vi "Read Config File (SubVI).vi"(0 "configuration file path":path=path "C:/Projet_CETAL_DESY_CSCI/POSTES LOCAUX/PROJECT_GAIA_HP/Development/Config/User.ini" caption="chemin du fichier de configuration", 5 "entrée d'erreur (pas d'erreur)":errorcluster) -> (14 "file path":path, 15 "User file contents Watlow":dbl[](array[numeric]), 18 "error?":bool caption="erreur ?", 19 "sortie d'erreur":errorcluster)   [LabVIEW 2017]
doc: "by Tanguy BOULARD"
uses:
  <vilib>/Utility/config.llb/Read Key (String).vi
  <vilib>/Utility/config.llb/NI_LVConfig.lvlib
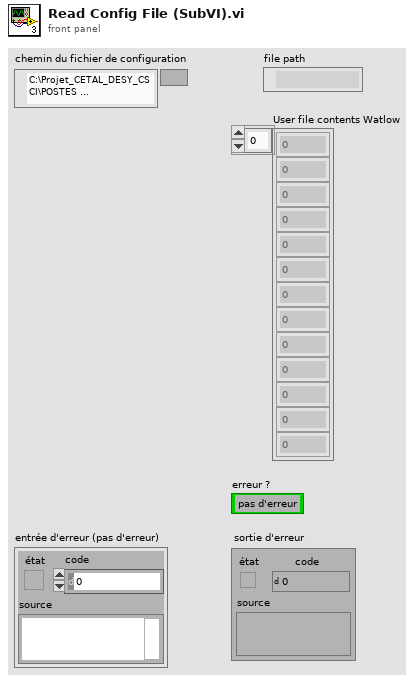
[diagram p1: front panel]
types:
  T1 = typedef "NI_LVConfig.lvlib/Config Data RefNum.ctl" = refnum<k1>
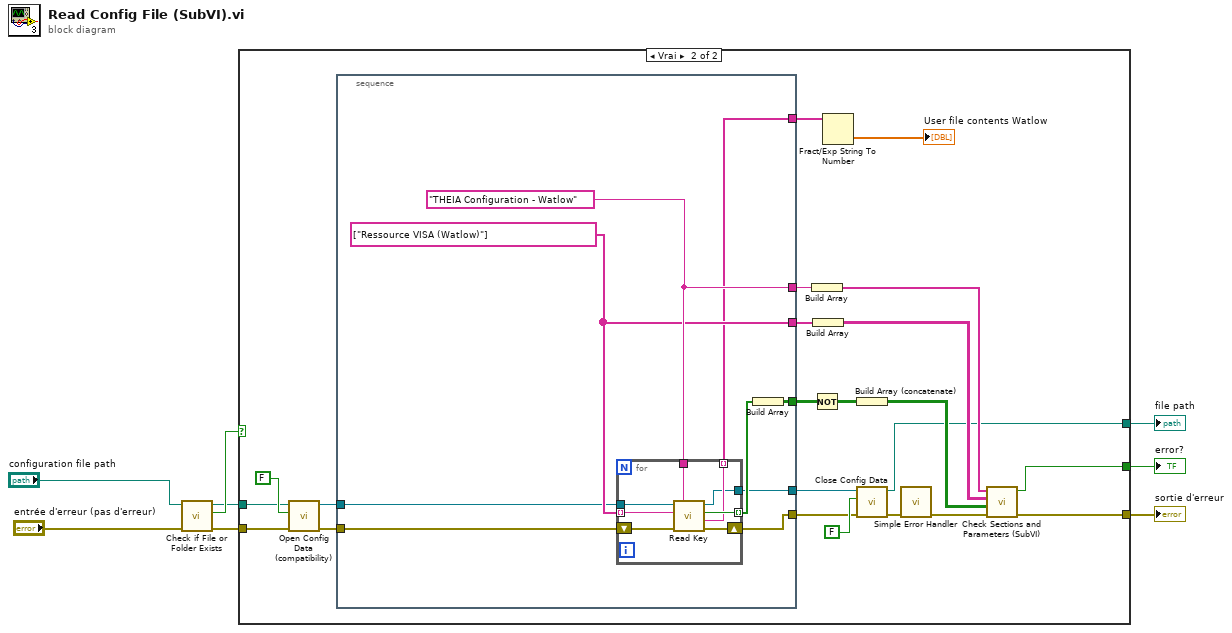
[diagram p0: block diagram]
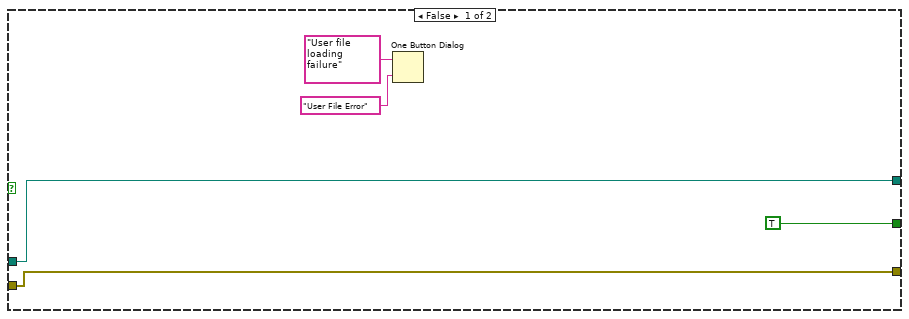
[diagram p2: hidden frame]
diagram:
  n1 = call <vilib>:"Check if File or Folder Exists.vi"("error in (no error)"="entrée d'erreur (pas d'erreur)", "path"="configuration file path") -> ("error out"=w5:errorcluster, "file or folder exists?"=w8:bool, "dup path"=w6:path)  [unwired: 7 in]
  n2 = case shown="Vrai" w8 {
    tunnel: w6 -> [w9 w31]
    tunnel: w5 -> [w11 w28]
    tunnel: [w11 w23] -> w3
    tunnel: [TRUE ("Erreur ?") w22] -> w4
    tunnel: [w9 w15] -> w1
    frame False {
      n3 = One Button Dialog(message="User file loading failure" ("Line1_message"), button name ("OK")="User File Error" ("Title")) -> ()  [unwired: 1 out]
    }
    frame True {
      n4 = call <vilib>:"Open Config Data (compatibility).vi"("error in (no error)"=w28, "create file if necessary (T)"=FALSE ("create file if necessary? (T)"), "configuration file path"=w31) -> ("error out"=w34:errorcluster, "refnum"=w29:T1)  [unwired: 6 in, 1 out]
      n5 = stacked-sequence {
        tunnel: w34 -> [w44]
        tunnel: w29 -> [w40]
        tunnel: [w37] -> w30
        tunnel: [w43] -> w27
        tunnel: [w41] -> w26
        tunnel: [w38] -> w25
        tunnel: [w39] -> w16
        tunnel: [w36] -> w14
        frame #0 {
          w41 = string[] ["Ressource VISA (Watlow)"]
          w43 = "THEIA Configuration - Watlow" ("section")
          n6 = for {
            shift-right: [w51] -> w37
            shift-left: w44 -> [w52]
            tunnel: w43 -> [w50]
            tunnel: w41 -> [w49] mode=indexing
            tunnel: w40 -> [w48]
            tunnel: [w47] -> w42 mode=indexing
            tunnel: [w46] -> w39 mode=indexing
            tunnel: [w45] -> w36
            n7 = call-poly <vilib>:"Read Key.vi"("section"=w50, "error in (no error)"=w52, "key"=w49, "refnum"=w48) -> ("error out"=w51:errorcluster, "value"=w46:string, "found?"=w47:bool, "refnum out"=w45:T1)  [unwired: 2 in, 2 out]
          }
          n8 = Build Array(w42) -> (w38:bool[][])
        }
      }
      n9 = Build Array(w27) -> (w21:string[])
      n10 = Not(x=w25) -> (.not. x?=w24:bool[][])
      n11 = Build Array(w26) -> (w20:string[][])
      n12 = Fract/Exp String To Number(string=w16) -> (number=→"User file contents Watlow":dbl[])  [unwired: 3 in, 1 out]
      n13 = Build Array (concatenate)(w24) -> (w19:bool[][])
      n14 = call <vilib>:"Close Config Data.vi"("error in (no error)"=w30, "write file if changed (T)"=FALSE ("write configuration file? (T)"), "refnum"=w14) -> ("error out"=w33:errorcluster, "file path"=w15:path)  [unwired: 7 out]
      n15 = call <vilib>:"Simple Error Handler.vi"("error in (no error)"=w33) -> ("error out"=w18:errorcluster)  [unwired: 1 in, 7 out]
      n16 = call "Check Sections and Parameters (SubVI).vi"("entrée d'erreur (pas d'erreur)"=w18, "found? array"=w19, "Parameter array"=w20, "Section array"=w21) -> ("sortie d'erreur"=w23:errorcluster, "Erreur ?"=w22:bool)  [unwired: 6 in]
    }
  }
  "error?" <- w4
  "sortie d'erreur" <- w3
  "file path" <- w1
